vi "Get Sheet Name (Idx).vi"(7 "Sheet":i32, 8 "error in (no error)":errorcluster, 11 "Workbook Reference":refnum<k24>) -> (0 "error out":errorcluster, 3 "Workbook Reference":refnum<k24>, 6 "Sheet Name (Sheet1)":string="Sheet1")   [LabVIEW 2013]
uses:
  C:/PhaeronGit/LVNPOI/Resources/NPOI 2.1.1 dotnet2/NPOI.dll
  Resources/NPOI 2.1.1 dotnet2/NPOI.dll
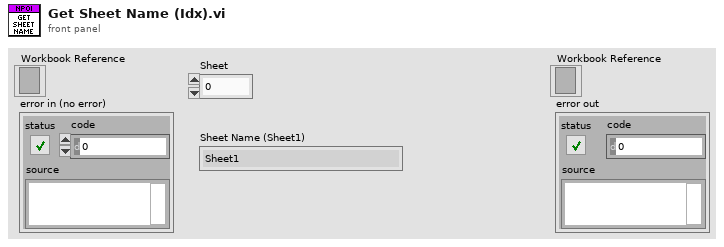
[diagram p1: front panel]
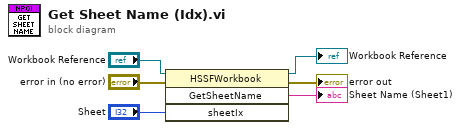
[diagram p0: block diagram]
diagram:
  n1 = invoke class="HSSFWorkbook" method="GetSheetName"(reference="Workbook Reference", error in="error in (no error)", "sheetIx"="Sheet") -> (reference out=→"Workbook Reference":refnum<k24>, error out=→"error out":errorcluster, "GetSheetName"=→"Sheet Name (Sheet1)":string)  [unwired: 1 in, 1 out]
